vi "Target Pose.vi"() -> ()   [LabVIEW 2017]
panel:
  in  "Target Y (Relative)":dbl
  in  "Target X (Relative)":dbl
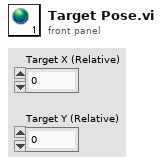
[diagram p1: front panel]
diagram:
